vi "Teardown.vi"(7 "Sender":refnum<class "Sender.lvclass">, 11 "Base jettl in":refnum<class "Base jettl.lvclass">) -> (3 "Base jettl out":refnum<class "Base jettl.lvclass">)   [LabVIEW 2021, in "jettl.lvlib" / "Base jettl.lvclass"]
uses:
  Base jettl.lvclass
  Sender/Sender/Sender.lvclass
  State.ctl
  Base jettl.lvclass/Base jettl.ctl
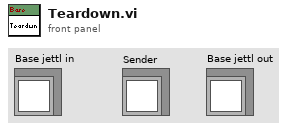
[diagram p1: front panel]
types:
  T1 = typedef "jettl.lvlib/Base jettl.lvclass/State.ctl" = enum16{"Nominal", "Teardown", "Error"}
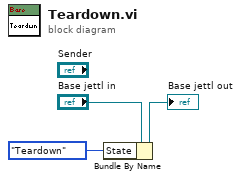
[diagram p0: block diagram]
diagram:
  n1 = Bundle By Name(cluster="Base jettl in", "State"=State."Teardown") -> (→"Base jettl out":refnum<class "Base jettl.lvclass">)
